vi "Close.vi"(8 "error in (no error)":errorcluster, 11 "1553 Board in":refnum<class "1553 Session.lvclass">) -> (0 "error out":errorcluster)   [LabVIEW 2020, in "BCI-1553 API.lvlib" / "1553 Session.lvclass"]
doc: "Closes all the references and sessions opened by the 1553 Session. It is recommended to call the 'Stop' method before calling this if a 1553 Session was started."
uses:
  1553 Session.lvclass
  1553 Session.lvclass/1553 Session.ctl
  1553 Component/1553 Component.lvclass
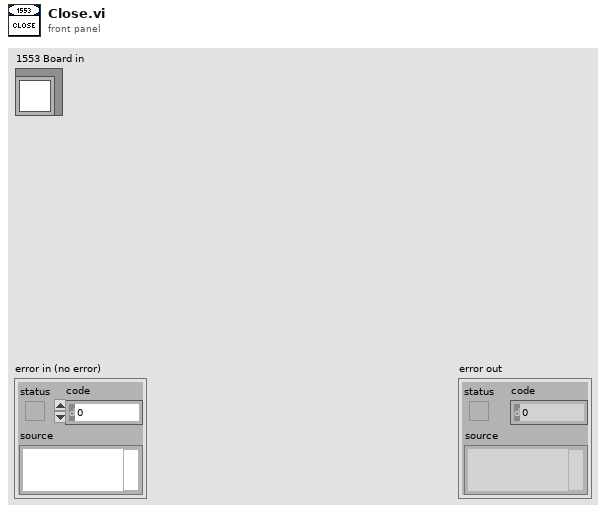
[diagram p1: front panel]
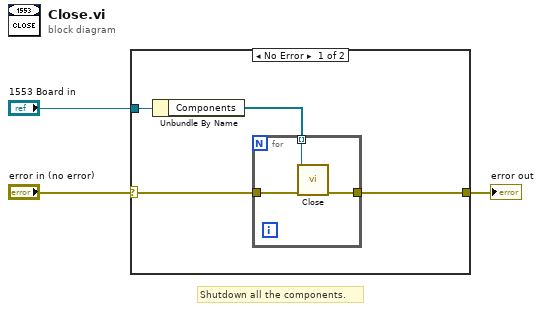
[diagram p0: block diagram]
diagram:
  # "Shutdown all the components."
  n1 = case shown="No Error" "error in (no error)" {
    selector: "error in (no error)" -> [w4 w11]
    tunnel: [w6 w11] -> w2
    tunnel: "1553 Board in" -> [w7 _]
    frame No Error {
      n2 = Unbundle By Name(w7) -> ("Components"=w5:refnum<class "1553 Component.lvclass">[])
      n3 = for {
        tunnel: w4 -> [w8]
        tunnel: [w10] -> w6
        tunnel: w5 -> [w9] mode=indexing
        n4 = call-dynamic "Close.vi"("error in (no error)"=w8, "1553 Component in"=w9) -> ("error out"=w10:errorcluster)  [unwired: 9 in]
      }
    }
    frame Error {
    }
  }
  "error out" <- w2
